vi "FGV - Nest Data Cache.vi"(8 "Error In":errorcluster, 9 "Nest Data":string, 10 "Nest Data FGV State":T1) -> (0 "Error Out":errorcluster, 2 "Nest Cached Data":string)   [LabVIEW 2013, in "LMH-Nest.lvlib"]
doc: "FGV used to cache Nest data. This allows values to be extracted without querying the Nest server."
uses:
  LMH-Nest.lvlib
  Type Defs/Nest Data FGV State.ctl
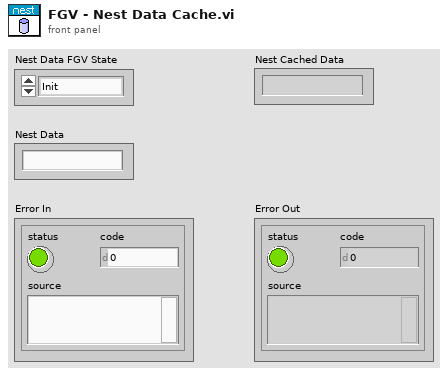
[diagram p1: front panel]
types:
  T1 = typedef "LMH-Nest.lvlib/Nest Data FGV State.ctl" = enum16{"Init", "Set", "Get"}
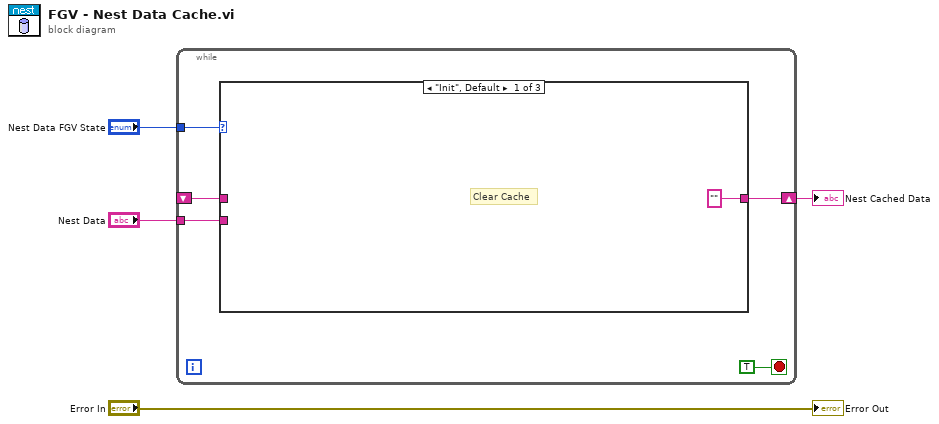
[diagram p0: block diagram]
diagram:
  n1 = while {
    tunnel: "Nest Data FGV State" -> [w8]
    shift-right: [w7] -> w3
    shift-left: _ -> [w5]
    tunnel: "Nest Data" -> [w6]
    stop <- TRUE stop-if-true
    n2 = case shown="\"Init\", Default" w8 {
      tunnel: ["" w11 w12] -> w7
      tunnel: w6 -> [_ w11 _]
      tunnel: w5 -> [_ _ w12]
      frame "Init", Default {
        # "Clear Cache"
      }
      frame "Set" {
      }
      frame "Get" {
      }
    }
  }
  "Nest Cached Data" <- w3
  "Error Out" <- "Error In"
